vi "FPGA LED.vi"   [LabVIEW 2016]
uses:
  <vilib>/rvi/Emulation/niFpgaGetClockAttributes.vi
  <vilib>/rvi/Emulation/niFpgaSctlEmulationGetInTimedLoop.vi
  <vilib>/rvi/Emulation/niFpgaEmulationReportErrorSimple.vi
  <vilib>/rvi/DataTransferAndStorage/Container/Common/niFpgaContainerExecOnDevCompGetState.vi
  <vilib>/rvi/Emulation/niFpgaEmulationIsFPGAContextNoSignature.vi
  <vilib>/rvi/errors/niFpgaSetErrorForExecOnDevCompSimple.vi
  <vilib>/rvi/eio/common/nirviEmuReportErrorAndStop.vi
  <vilib>/rvi/DataTransferAndStorage/Container/Common/niFpgaContainerGetUniqueNameForEmu.vi
  <vilib>/rvi/FIFO/Fifo_Resource/nirvififoEmulationSetSize.vi
  <vilib>/rvi/FIFO/Fifo_Resource/nirviFifoEmulationQueueMgr.vi
  <instcachedir>/0/nirviFifoEmulationQueueMgr_E5CAEC123FF24DC58D834DCA3CDAA9B5.lvgen/nirviFifoEmulationQueueMgr_E5CAEC123FF24DC58D834DCA3CDAA9B5_003.vi
  <vilib>/rvi/FIFO/Fifo_Resource/nirvififoEmulationDetermineInputValidOut.vi
  <vilib>/rvi/FIFO/Fifo_Resource/nirvififoEmulationCreateLock.vi
  <vilib>/rvi/Emulation/niFpgaProcessEmulError.vi
  <vilib>/rvi/FIFO/Fifo_Resource/nirvififoEmulationObtainLock.vi
  <vilib>/rvi/FIFO/Fifo_Resource/nirvififoEmulationReleaseLock.vi
  <vilib>/rvi/occurrence/nirviWaitOnOccurrenceBase.vi
  <vilib>/rvi/errors/nirviReportUnexpectedCaseInternalError.vi
  <vilib>/rvi/errors/nirviReportUnexpectedCaseInternalError (U32).vi
  <vilib>/Utility/error.llb/Clear Errors.vi
  <vilib>/rvi/interface/RandomDataEmulation/niFpgaRandomDataHandleErrors.vi
  <vilib>/rvi/eio/common/nirviEmuTemplateMethod_errors.vi
  <vilib>/rvi/Emulation/niFpgaCriticalErrorInLSC.vi
  <vilib>/rvi/DataTransferAndStorage/Container/XNode/niFpgaContainer.xnode
  <vilib>/rvi/FIFO/Fifo_Resource/niFpgaFifoEmulationRefIn.vi
  <vilib>/eio/EIONode/EIONode.xnode
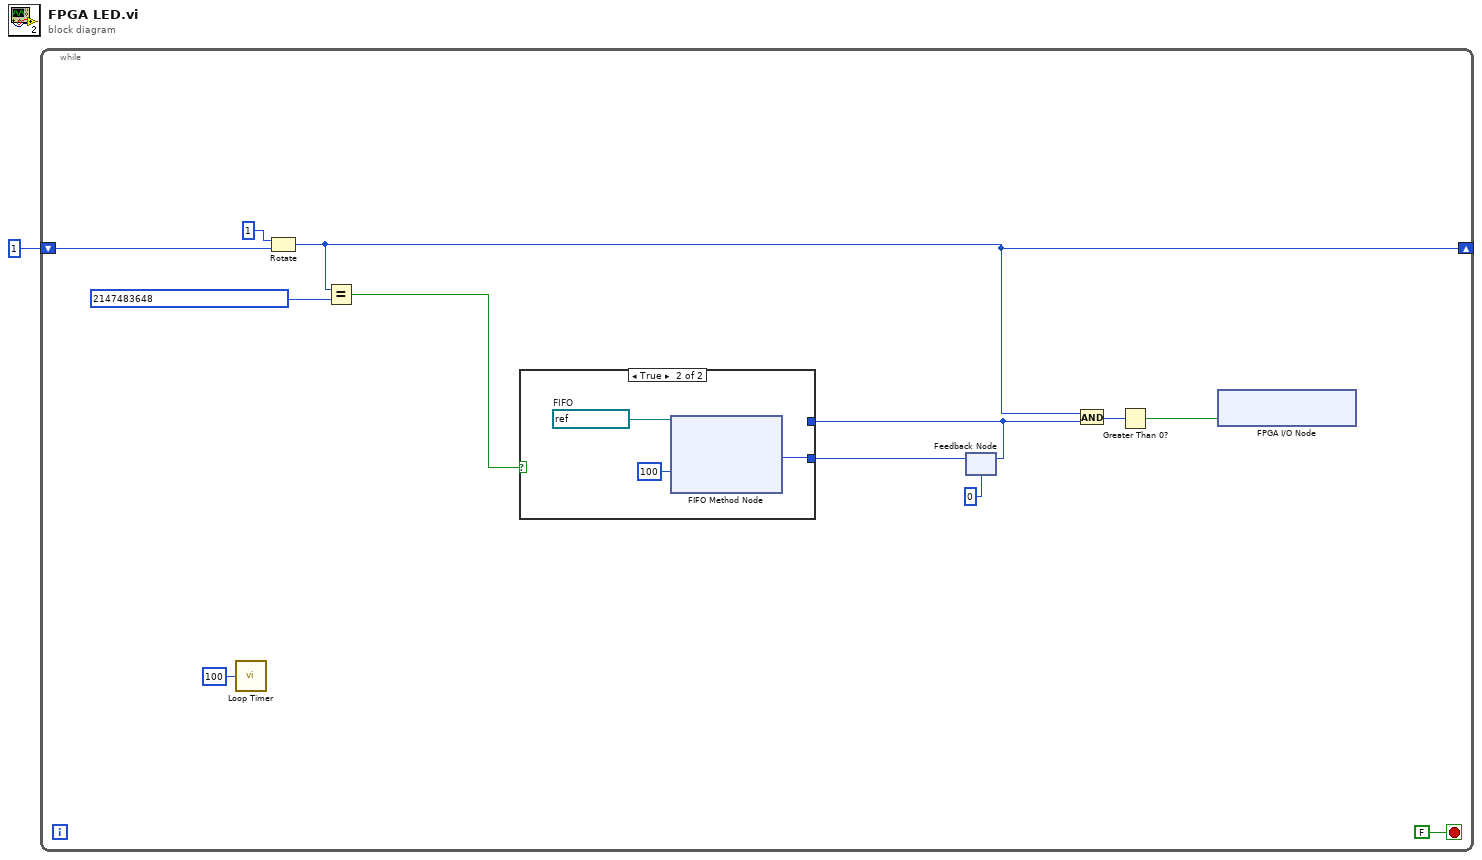
[diagram p0: block diagram]
diagram:
  n1 = while {
    shift-right: [w5] -> _
    shift-left: u32 1 -> [w7]
    stop <- FALSE stop-if-true
    n2 = call "Loop Timer"("Count(mSec)"=u32 100) -> ()  [unwired: 1 out]
    n3 = Rotate(1:w7, 2:i16 1 ("y")) -> (0:w5:u32)
    n4 = Equal?(x=w5, y=u32 2147483648) -> (x = y?=w11:bool)
    n5 = feedback #1(u32 0 ("Element")) -> (w3:u32)
    n6 = case shown="True" w11 {
      tunnel: [w14 w15] -> w4
      tunnel: w3 -> [w14 _]
      frame False {
      }
      frame True {
        w17 = refnum<k21> "LED_FIFO"  # FIFO
        n7 = xnode ("FIFO Method Node")("Timeout"=100, "FIFO In"=w17) -> ("Element"=w15:u32)  [unwired: 2 out]
      }
    }
    n8 = feedback-in #1(w4) -> ()
    n9 = And(x=w5, y=w3) -> (x .and. y?=w9:u32)
    n10 = Greater Than 0?(x=w9) -> (x > 0?=w8:bool)
    n11 = xnode "FPGA I/O Node"("ConnectorC/DIO0"=w8) -> ()  [unwired: 1 in, 1 out]
  }
